vi "Write ch_units.vi"(8 "error in (no error)":errorcluster, 10 "ch_units":string[](array[string]), 11 "launcher in":refnum<class "launcher.lvclass">) -> (0 "error out":errorcluster, 3 "launcher out":refnum<class "launcher.lvclass">)   [LabVIEW 2021, in "launcher.lvclass"]
uses:
  launcher.lvclass
  launcher.lvclass/launcher.ctl
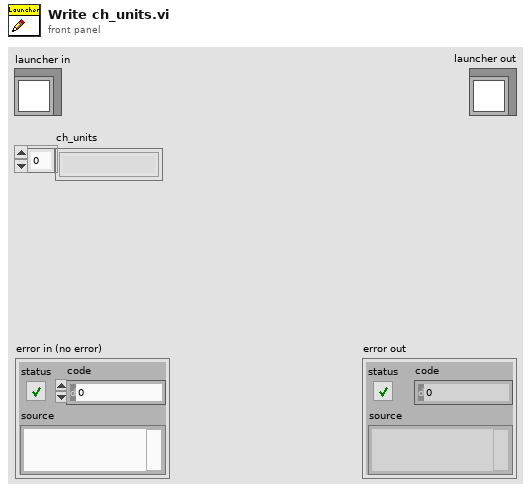
[diagram p1: front panel]
types:
  T1 = typedef "launcher.lvclass/dvr_type.ctl" = cluster{"_PARMS":T2}
  T2 = typedef "launcher.lvclass/_PARMS.ctl" = cluster{"ch_alias":string[], "ch_units":string[], "Modules to Launch":T3[]}
  T3 = typedef "Module.lvclass/Launch Module Typdef.ctl" = cluster{"Module":string, "Parameters":T4}
  T4 = typedef "Module.lvclass/Launch Module Parms.ctl" = cluster{"Name":string, "Arguments":string[], "Show FP?":bool}
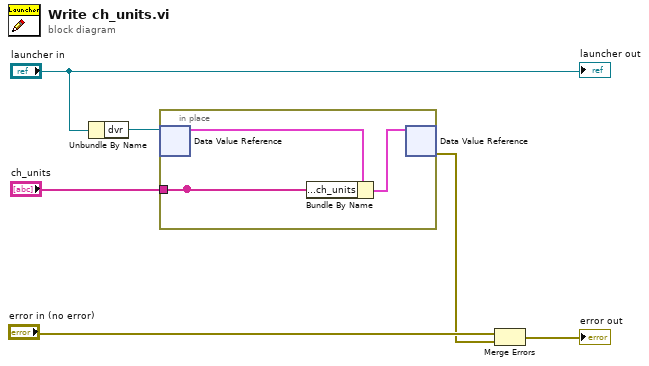
[diagram p0: block diagram]
diagram:
  n1 = Unbundle By Name ("DVR Unbundle")("launcher in") -> ("dvr"=w2:refnum<data-value>)
  n2 = in-place "In Place Element Structure" {
    in-place-border: [w7] -> _
    in-place-border: "ch_units" -> [w7]
    n3 = in-place-dvr #1(w2) -> (w9:T1)  [unwired: 1 out]
    n4 = Bundle By Name ("Item Bundle")(cluster=w9, "_PARMS.ch_units"=w7) -> (w8:T1)
    n5 = in-place-dvr #1(w8) -> (w3:errorcluster)  [unwired: 1 out]
  }
  n6 = Merge Errors("error in (no error)", w3) -> (→"error out":errorcluster)
  "launcher out" <- "launcher in"
